vi "Read_Encoders_v2.vi"(8 "error in (no error)":errorcluster, 10 "Cluster in":T3={FALSE, "Tick Count(uSec)"=0, "Counter Value"=[0, 0, 0, 0], "x-y"=[0, 0, 0, 0]}, 11 "Encoder 1 Controller":T2={"Sample time (uS)"=300000, "Reset"=FALSE}) -> (0 "error out":errorcluster, 1 "Cluster Out":T3, 2 "Updated":bool, 3 "appended array":i64[](array[numeric]), 4 "Output Cluster":T1, 5 "Tick Count(uSec)":u32 caption="Tick Count(Ticks)")   [LabVIEW 2018]
uses:
  <vilib>/rvi/Arithmetic/AddSubMult/XNode/nirviSatArithmetic.xnode
  <vilib>/Studica/Studica Toolkit/Background/Mxp Selection.ctl
  EuroSkills Budapest 2018/Robotiikka21.12/Robotiikka/Controls/EncoderController.ctl
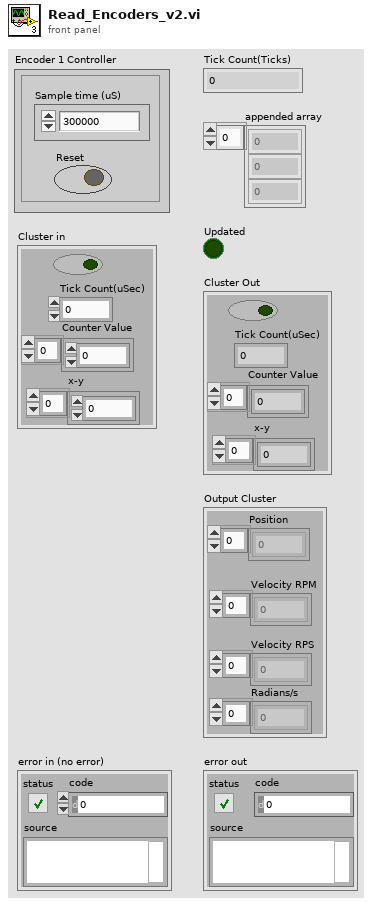
[diagram p1: front panel]
types:
  T1 = cluster{"Position":i32[], "Velocity RPM":dbl[], "Velocity RPS":dbl[], "Radians/s":dbl[]}
  T2 = typedef "EncoderController.ctl" = cluster{"Sample time (uS)":u32, "Reset":bool}
  T3 = cluster{bool, "Tick Count(uSec)":u32, "Counter Value":i32[], "x-y":i32[]}
  T4 = typedef "Mxp Selection.ctl" = enum16{"MXP A", "MXP B"}
  T5 = cluster{bool, "Tick Count(uSec)":u32, "Counter Value":dbl[], "x-y":dbl[]}
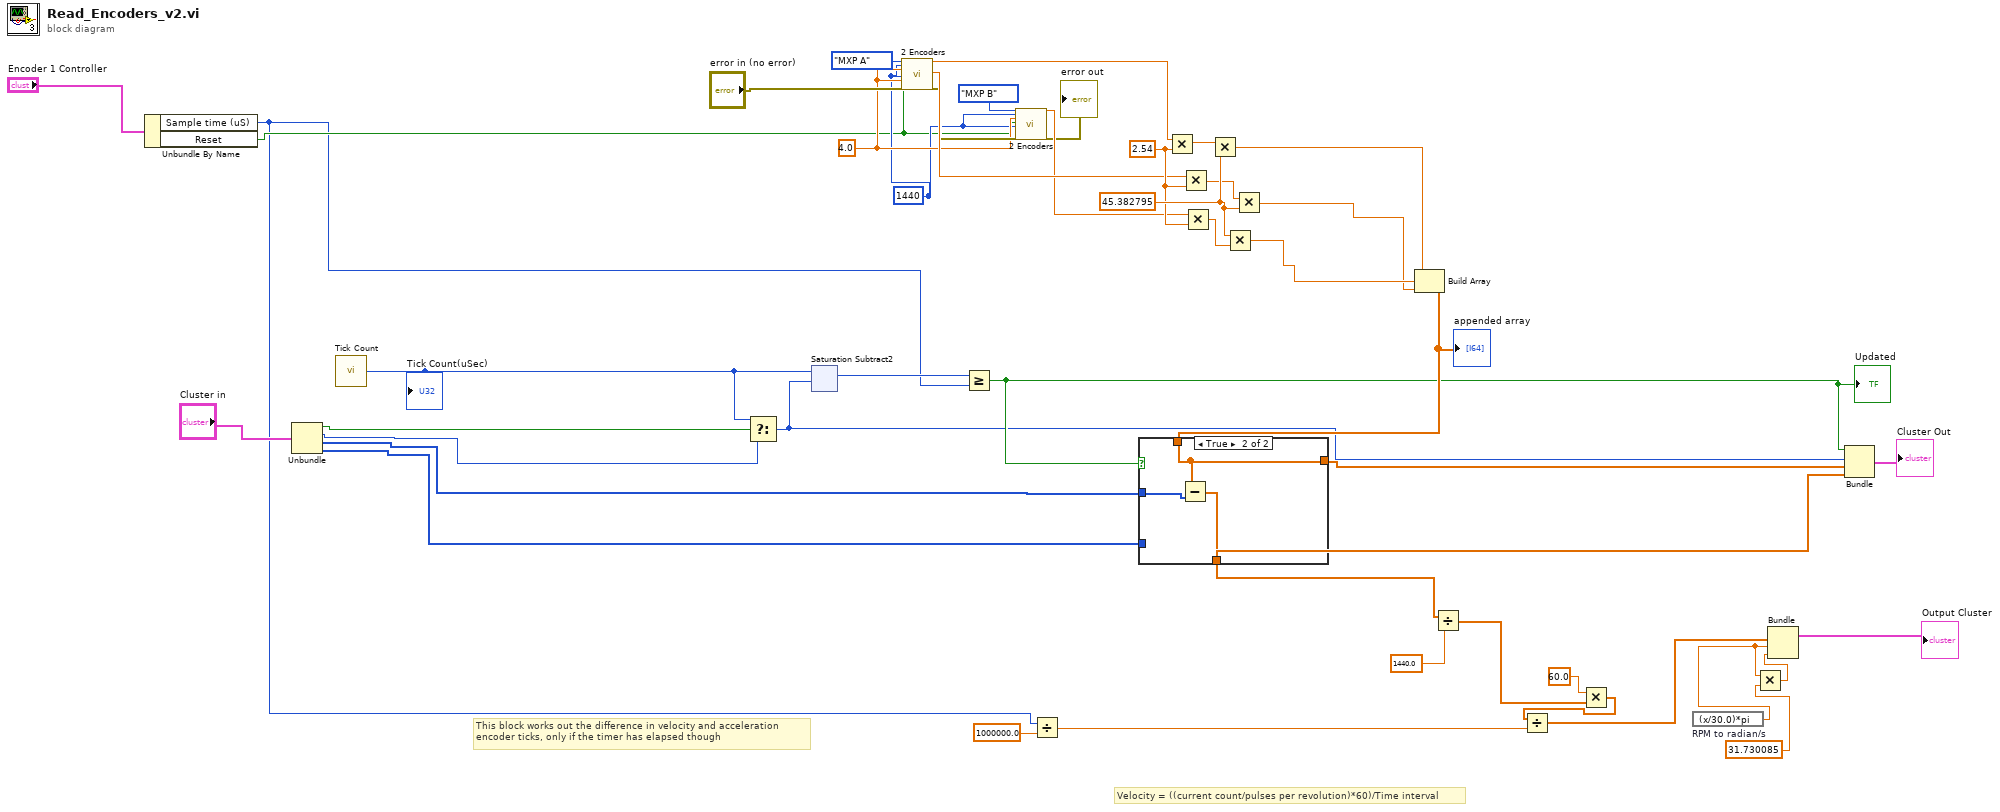
[diagram p0: block diagram]
diagram:
  w36 = 45.382795 ("y")
  w9 = 4.0 ("Wheel Diameter M1 (inches)")
  w8 = u32 1440 ("Ticks Per Rev M0")
  w18 = 2.54 ("y")
  # "Velocity = ((current count/pulses per revolution)*60)/Time interval"
  # "This block works out the difference in velocity and acceleration \nencoder ticks, only if the timer has elapsed though"
  n1 = Unbundle By Name("Encoder 1 Controller") -> ("Sample time (uS)"=w5:u32, "Reset"=w6:bool)
  n2 = Unbundle("Cluster in") -> (w30:bool, "Tick Count(uSec)"=w31:u32, "Counter Value"=w32:i32[], "x-y"=w33:i32[])
  n3 = call "Tick Count"() -> ("Tick Count(uSec)"=w21:u32)
  "Tick Count(uSec)" <- w21
  n4 = Select(t=w21, s=w30, f=w31) -> (s? t:f=w22:u32)
  n5 = xnode ("Saturation Subtract2")("x"=w21, "y"=w22) -> ("x-y"=w26:u32)
  n6 = call <vilib>:"2 Encoders.vi"("Mxp Side"=Mxp_Selection."MXP A", "Ticks Per Rev M0"=w8, "Wheel Diameter M0 (inches)"=w9, "Reset Encoder 0"=w6, "Ticks Per Rev M1"=w8, "Wheel Diameter M1 (inches)"=w9, "Reset Encoder 1"=w6, "error in (no error)"="error in (no error)") -> ("Distance M0 (inches)"=w17:dbl, "Distance M1 (inches)"=w16:dbl, "error out"=w13:errorcluster)  [unwired: 17 in]
  n7 = Greater Or Equal?(x=w26, y=w5) -> (x >= y?=w23:bool)
  "Updated" <- w23
  n8 = call <vilib>:"2 Encoders.vi"("Mxp Side"=Mxp_Selection."MXP B", "Ticks Per Rev M0"=w8, "Wheel Diameter M0 (inches)"=w9, "Reset Encoder 0"=w6, "Ticks Per Rev M1"=w8, "error in (no error)"=w13) -> ("Distance M0 (inches)"=w15:dbl, "error out"=→"error out":errorcluster)  [unwired: 19 in, 1 out]
  n9 = Divide(x=w5, y=1000000.0) -> (x/y=w1:dbl)
  n10 = Multiply(x=w17, y=w18) -> (x*y=w34:dbl)
  n11 = Multiply(x=w16, y=w18) -> (x*y=w35:dbl)
  n12 = Multiply(x=w15, y=w18) -> (x*y=w37:dbl)
  n13 = Multiply(x=w34, y=w36) -> (x*y=w38:dbl)
  n14 = Multiply(x=w36, y=w37) -> (x*y=w40:dbl)
  n15 = Multiply(x=w35, y=w36) -> (x*y=w39:dbl)
  n16 = Build Array(w38, w40, w39) -> (w27:dbl[])
  "appended array" <- w27
  n17 = case shown="True" w23 {
    tunnel: w32 -> [w46 w50]
    tunnel: [w47 w49] -> w42
    tunnel: w33 -> [w47 _]
    tunnel: [w46 w48] -> w20
    tunnel: w27 -> [_ w48]
    frame False {
    }
    frame True {
      n18 = Subtract(x=w48, y=w50) -> (x-y=w49:dbl[])
    }
  }
  n19 = Divide(x=w42, y=1440.0) -> (x/y=w3:dbl[])
  n20 = Multiply(x=60.0 ("y"), y=w3) -> (x*y=w2:dbl[])
  n21 = Divide(x=w2, y=w1) -> (x/y=w7:dbl[])
  n22 = expression code="(x/30.0)*pi" "RPM to radian/s"() -> (w41:dbl)  [unwired: 1 in]
  n23 = Multiply(x=w41, y=31.730085) -> (x*y=w44:dbl)
  n24 = Bundle(w7, w41, w44) -> (→"Output Cluster":cluster{void, dbl[], dbl, dbl})  [unwired: 2 in]
  n25 = Bundle(w23, "Tick Count(uSec)"=w22, "Counter Value"=w20, "x-y"=w42) -> (→"Cluster Out":T5)  [unwired: 1 in]
